vi "niDDC Configure Channels.vi"(8 "error in (no error)":errorcluster, 10 "mode":T1(ring)=enum."TIS mode (CH0 only)", 11 "Class in":refnum<class "7976R_v1.lvclass">) -> (0 "error out":errorcluster, 3 "Class out":refnum<class "7976R_v1.lvclass">)   [LabVIEW 2015, in "7976R_v1.lvclass"]
uses:
  <userlib>/SE-APP-Receiver/NI5772/7976R_v1/7976R_v1.lvclass
  <userlib>/SE-APP-Receiver/NI5772/7976R_v1/Private/TIS Mode_v1.ctl
  <userlib>/SE-APP-Receiver/NI5772/7976R_v1/7976R_v1.lvclass/7976R_v1.ctl
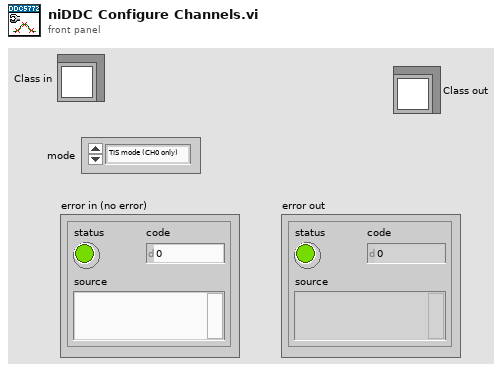
[diagram p1: front panel]
types:
  T1 = enum16{"Normal mode", "TIS mode (CH0 only)", "TIS mode (CH1 only)"}
  T2 = typedef "7976R_v1.lvclass/TIS Mode_v1.ctl" = u16
  T3 = typedef "7976R_v1.lvclass/FPGA VI Reference_DDC_v1.8.ctl" = refnum<k20>
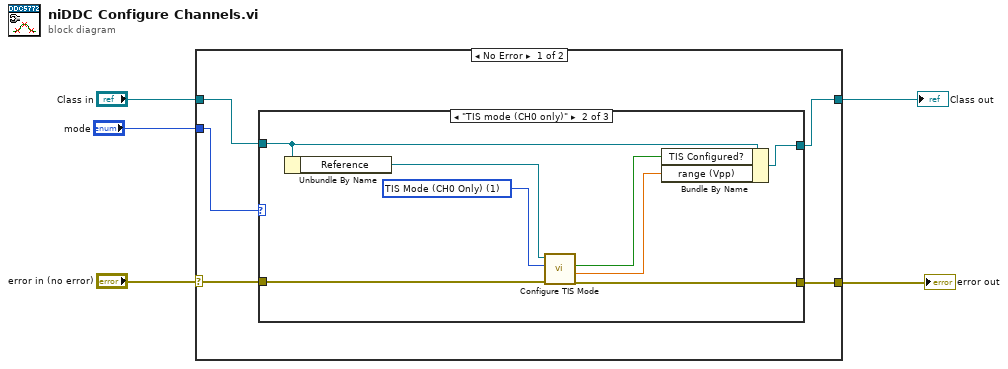
[diagram p0: block diagram]
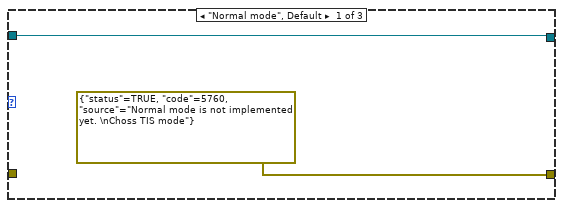
[diagram p2: hidden frame]
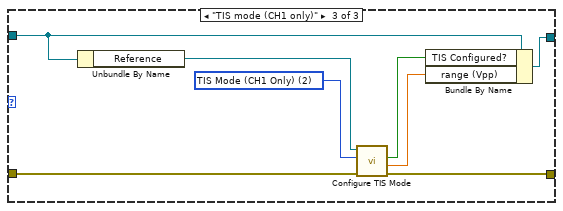
[diagram p3: hidden frame]
diagram:
  n1 = case shown="No Error" "error in (no error)" {
    selector: "error in (no error)" -> [w9 w29]
    tunnel: [w10 w29] -> w5
    tunnel: "mode" -> [w8 _]
    tunnel: "Class in" -> [w7 w30]
    tunnel: [w6 w30] -> w1
    frame No Error {
      n2 = case shown="\"TIS mode (CH0 only)\"" w8 {
        tunnel: [errorcluster {"status"=TRUE, "code"=5760, "source"="Normal mode is not implemented yet. \nChoss TIS mode"} ("error out") w19 w25] -> w10
        tunnel: w9 -> [_ w18 w26]
        tunnel: w7 -> [w11 w15 w24]
        tunnel: [w11 w16 w23] -> w6
        frame "Normal mode", Default {
        }
        frame "TIS mode (CH0 only)" {
          w20 = T2 1 items=["TIS Mode (CH0 Only)"=1, "TIS Mode (CH1 Only)"=2, "Dual TIS Mode (CH0 and CH1)"=3] ("TIS Mode")
          n3 = Unbundle By Name(w15) -> ("Reference"=w17:T3)
          n4 = call <userlib>:"Configure TIS Mode.vi"("error in"=w18, "TIS Mode"=w20, "Ref in"=w17) -> ("error out"=w19:errorcluster, "range (Vpp)"=w13:dbl, "TIS Configured?"=w14:bool)  [unwired: 5 in, 1 out]
          n5 = Bundle By Name(cluster=w15, "TIS Configured?"=w14, "range (Vpp)"=w13) -> (w16:refnum<class "7976R_v1.lvclass">)
        }
        frame "TIS mode (CH1 only)" {
          w28 = T2 2 items=["TIS Mode (CH0 Only)"=1, "TIS Mode (CH1 Only)"=2, "Dual TIS Mode (CH0 and CH1)"=3] ("TIS Mode")
          n6 = Unbundle By Name(w24) -> ("Reference"=w27:T3)
          n7 = call <userlib>:"Configure TIS Mode.vi"("error in"=w26, "TIS Mode"=w28, "Ref in"=w27) -> ("error out"=w25:errorcluster, "range (Vpp)"=w21:dbl, "TIS Configured?"=w22:bool)  [unwired: 5 in, 1 out]
          n8 = Bundle By Name(cluster=w24, "TIS Configured?"=w22, "range (Vpp)"=w21) -> (w23:refnum<class "7976R_v1.lvclass">)
        }
      }
    }
    frame Error {
    }
  }
  "error out" <- w5
  "Class out" <- w1
